vi "Test Laser Logicv.vi"() -> ()   [LabVIEW 2013]
panel:
  out "Numeric 2":i32
  out "Numeric":i32
  in  "Num2Acq":u16
  out "Waveform Chart":cluster{"Number of Samples":u16, i16}(graph)
  in  "Stop":bool
  in  "TotNumSamp":u16=1000
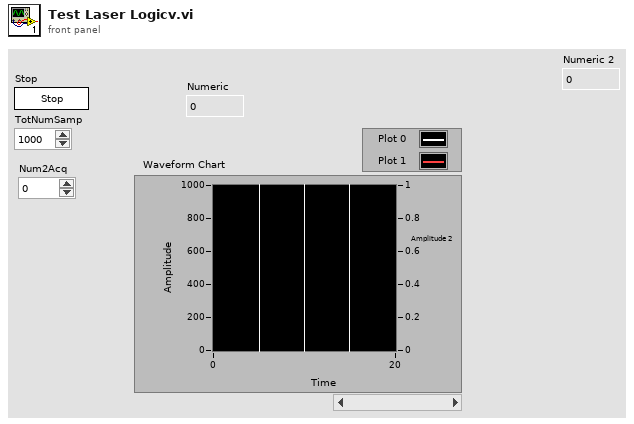
[diagram p1: front panel]
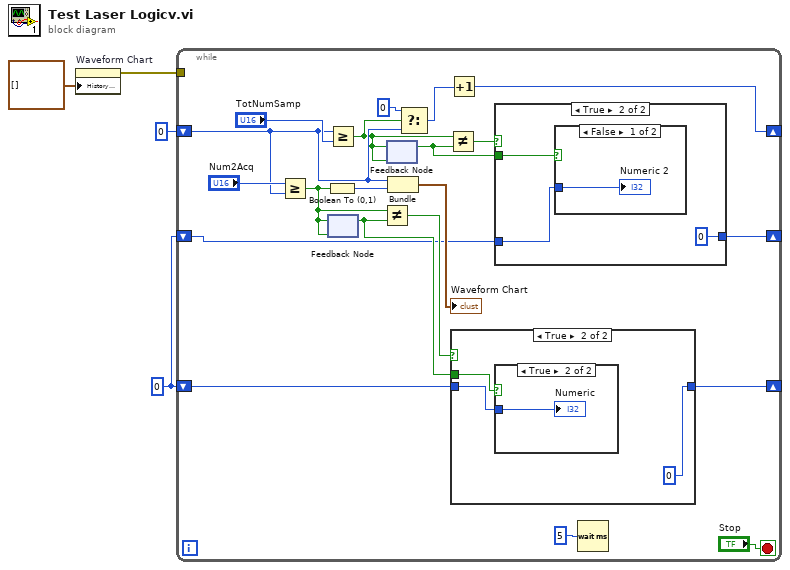
[diagram p0: block diagram]
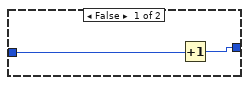
[diagram p2: hidden frame]
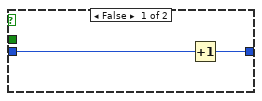
[diagram p4: hidden frame]
diagram:
  w2 = u16 0
  n1 = property on="Waveform Chart" class="WFChart (strict)"("History Data"=cluster{"Number of Samples":u16, i16}[] []) -> (error out=w3:errorcluster)  [unwired: 2 in, 1 out]
  n2 = while {
    shift-right: [w20] -> _
    shift-left: u16 0 -> [w16]
    tunnel: w3 -> [_]
    shift-right: [w11] -> _
    shift-left: w2 -> [w10]
    shift-right: [w6] -> _
    shift-left: w2 -> [w5]
    stop <- "Stop" stop-if-true
    n3 = Greater Or Equal?(x="Num2Acq", y=w16) -> (x >= y?=w14:bool)
    n4 = Boolean To (0,1)(Boolean=w14) -> (0, 1=w17:i16)
    n5 = Greater Or Equal?(x=w16, y="TotNumSamp") -> (x >= y?=w8:bool)
    n6 = feedback-in #1(w14) -> ()
    n7 = feedback #1(w14) -> (w12:bool)
    n8 = Not Equal?(x=w14, y=w12) -> (x != y?=w13:bool)
    n9 = feedback #2(w8) -> (w7:bool)
    n10 = feedback-in #2(w8) -> ()
    n11 = Bundle(w16, w17) -> (→"Waveform Chart":cluster{u16, i16})  [unwired: 1 in]
    n12 = Select(t=u16 0 ("Number of Samples"), s=w8, f=w16) -> (s? t:f=w21:u16)
    n13 = Not Equal?(x=w8, y=w7) -> (x != y?=w9:bool)
    n14 = Increment(x=w21) -> (x+1=w20:u16)
    n15 = case shown="True" w13 {
      tunnel: w12 -> [_ w35]
      tunnel: [w31 0] -> w11
      tunnel: w10 -> [w32 w33]
      frame False {
        n16 = Increment(x=w32) -> (x+1=w31:i32)
      }
      frame True {
        n17 = case shown="True" w35 {
          tunnel: w33 -> [_ w36]
          frame False {
          }
          frame True {
            "Numeric" <- w36
          }
        }
      }
    }
    n18 = case shown="True" w9 {
      tunnel: [w25 0] -> w6
      tunnel: w5 -> [w26 w28]
      tunnel: w7 -> [_ w27]
      frame False {
        n19 = Increment(x=w26) -> (x+1=w25:i32)
      }
      frame True {
        n20 = case shown="False" w27 {
          tunnel: w28 -> [w30 _]
          frame False {
            "Numeric 2" <- w30
          }
          frame True {
          }
        }
      }
    }
    n21 = Wait (ms)(milliseconds to wait=u32 5) -> ()  [unwired: 1 out]
  }
